vi "TCP.IP Server for Ripple Detection - Copy 3.vi"() -> ()   [LabVIEW 2021]
doc: "Demonstrates how to set up a basic TCP connection, send data to the specified port once a connection has been established, and terminate the connection once the data has been sent. This VI is designed to stop if the TCP connection is terminated. The data sent in this example is an array of random numbers."
panel:
  out "Waveform Graph 10":dbl[](graph)
  in  "loop 1":i32
  in  "Client Closed":string="The client VI closed the connection."
  in  "Stop":bool
  # "Overview: Demonstrates the use of the TCP functions to initialize a TCP server that can send data to a client VI.\nInstructions:\n1. Run the VI.\n2. Open Simple TCP - Client.vi and follow the instructions on its front panel. Note that if you wait longer than 30 seconds to do this after running this VI, it will time out.\n3. Click Stop to stop the VI. Note that if you stop the client VI, this VI will stop automatically."
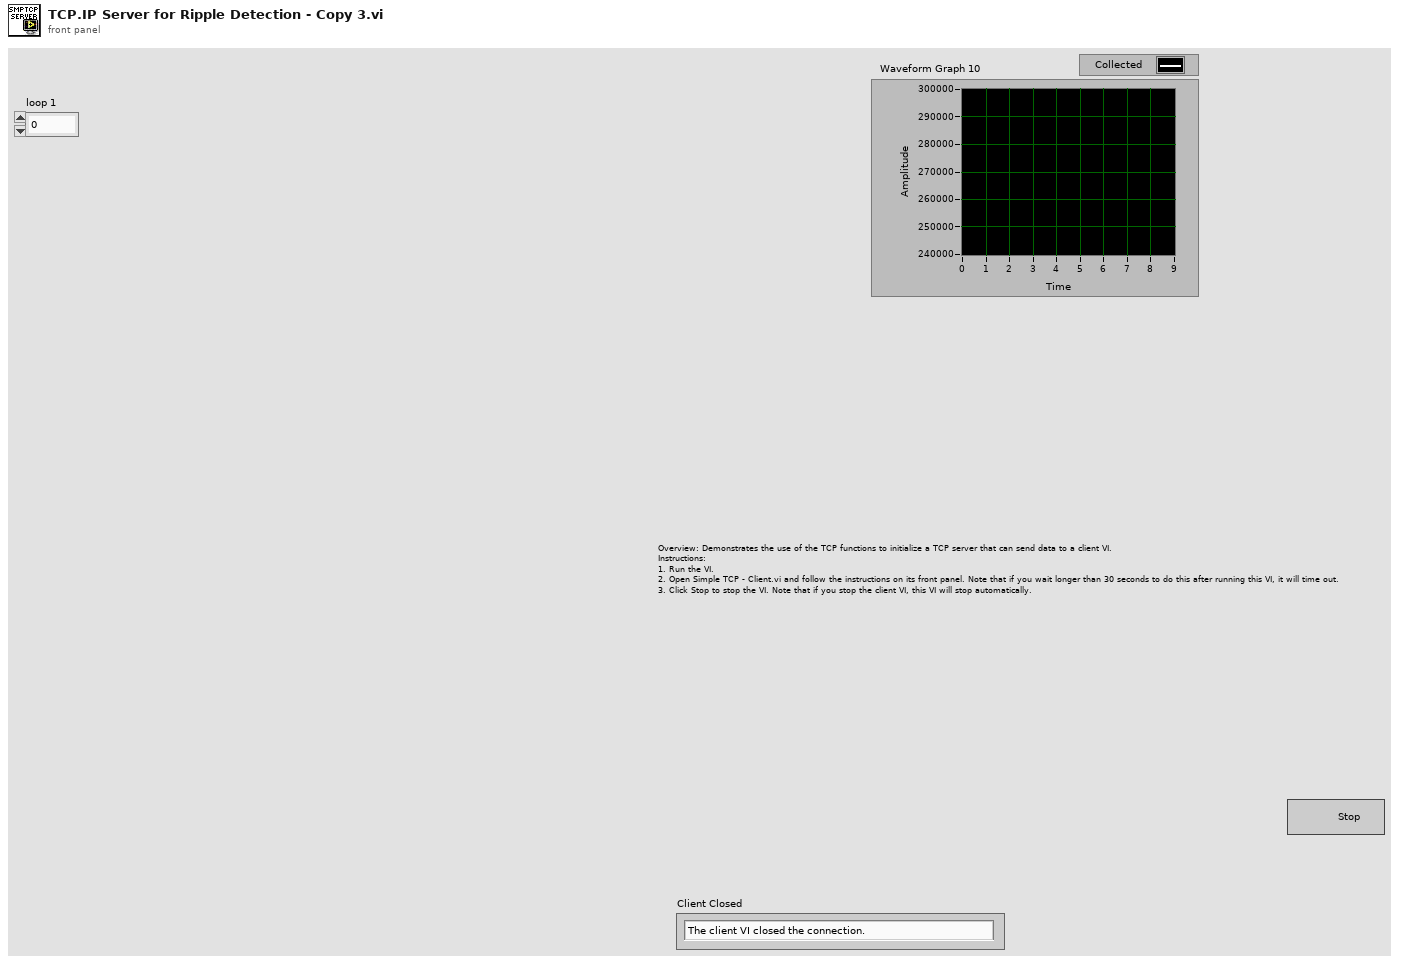
[diagram p1: front panel]
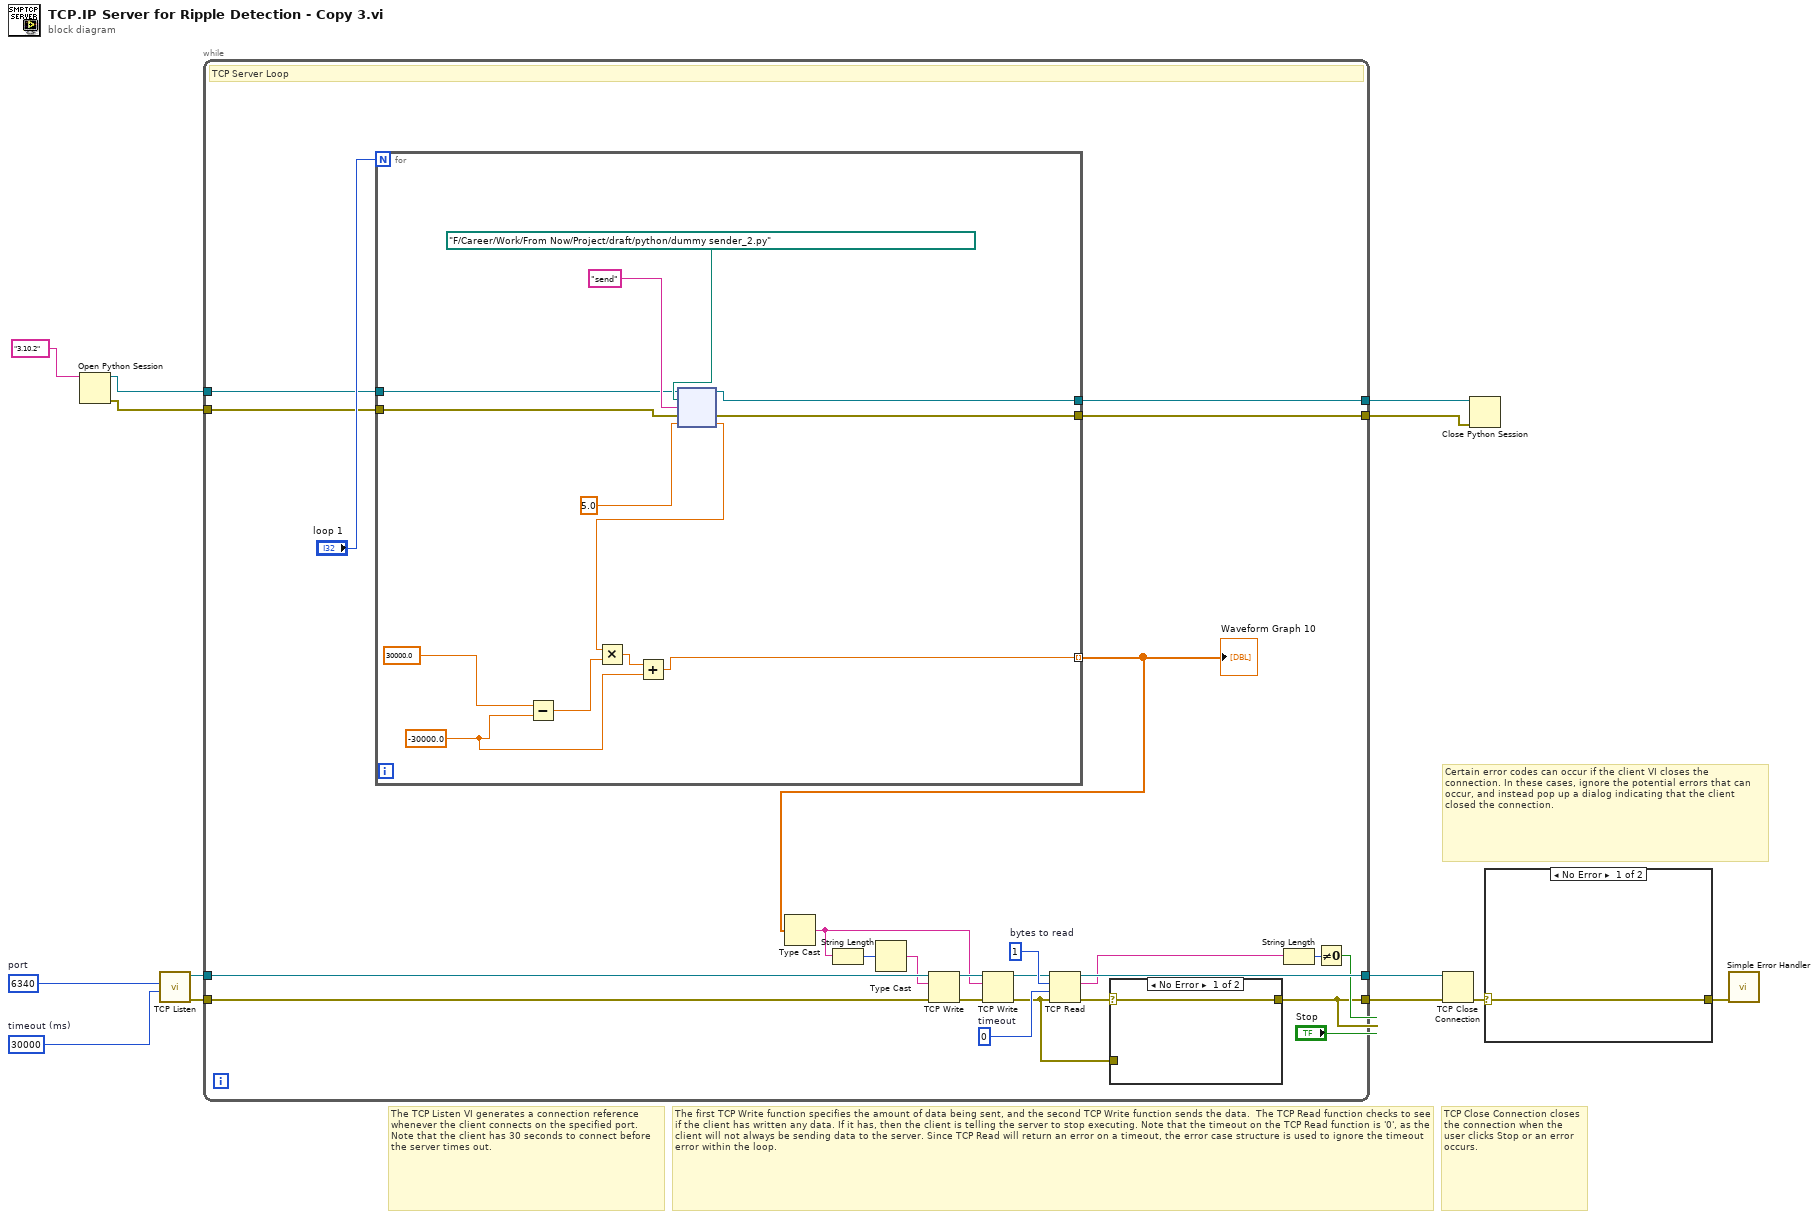
[diagram p0: block diagram]
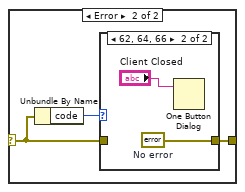
[diagram p2: hidden frame]
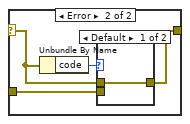
[diagram p4: hidden frame]
diagram:
  w6 = u16 6340  # port
  w7 = 30000  # timeout (ms)
  # "TCP Close Connection closes the connection when the user clicks Stop or an error occurs."
  # "The TCP Listen VI generates a connection reference whenever the client connects on the specified port. Note that the client has 30 seconds to connect before the server times out."
  # "Certain error codes can occur if the client VI closes the connection. In these cases, ignore the potential errors that can occur, and instead pop up a dialog indicating that the client closed the connection."
  # "The first TCP Write function specifies the amount of data being sent, and the second TCP Write function sends the data.  The TCP Read function checks to see if the client has written any data. If it has, then the client is telling the server to stop executing. Note that the timeout on the TCP Read function is '0', as the client will not always be sending data to the server. Since TCP Read will return an error on a timeout, the error case structure is used to ignore the timeout error within the loop."
  n1 = Open Python Session(python version="3.10.2" ("Python version")) -> (session out=w4:refnum<k35>, error out=w3:errorcluster)  [unwired: 2 in]
  n2 = call <vilib>:"TCP Listen.vi"("timeout ms (wait forever: -1)"=w7, "port"=w6) -> ("error out"=w8:errorcluster, "connection ID"=w9:refnum<k5>)  [unwired: 5 in, 3 out]
  n3 = while {
    tunnel: [w21] -> w12
    tunnel: [w27] -> w13
    tunnel: w9 -> [w38]
    tunnel: w8 -> [w31]
    tunnel: w4 -> [w17]
    tunnel: w3 -> [w16]
    tunnel: [w15] -> w2
    tunnel: [w14] -> w1
    stop <- w32 stop-if-true
    w26 = 0  # timeout
    w29 = 1  # bytes to read
    # "TCP Server Loop"
    n4 = for {
      N: "loop 1" -> [_]
      tunnel: [w43] -> w18 mode=indexing
      tunnel: w17 -> [w42]
      tunnel: w16 -> [w41]
      tunnel: [w40] -> w15
      tunnel: [w39] -> w14
      w48 = -30000.0 ("y")
      n5 = Subtract(x=30000.0, y=w48) -> (x-y=w51:dbl)
      n6 = node(w42, path "F:/Career/Work/From Now/Project/draft/python/dummy sender_2.py" ("module path"), "send" ("function name"), w41, 5.0) -> (w40:refnum<k35>, w39:errorcluster, w44:dbl)  [unwired: 2 out]
      n7 = Multiply(x=w44, y=w51) -> (x*y=w50:dbl)
      n8 = Add(x=w50, y=w48) -> (x+y=w43:dbl)
    }
    "Waveform Graph 10" <- w18
    n9 = Type Cast(x=w18) -> (*(type *) &x=w33:string)  [unwired: 1 out]
    n10 = String Length(string=w33) -> (length=w35:i32)
    n11 = Type Cast(x=w35) -> (*(type *) &x=w34:string)  [unwired: 1 out]
    n12 = TCP Write(connection ID=w38, data in=w34, error in (no error)=w31) -> (connection ID out=w37:refnum<k5>, error out=w36:errorcluster)  [unwired: 2 out]
    n13 = TCP Write(connection ID=w37, data in=w33, error in (no error)=w36) -> (connection ID out=w28:refnum<k5>, error out=w20:errorcluster)  [unwired: 2 out]
    n14 = TCP Read(connection ID=w28, bytes to read=w29, error in (no error)=w20, 9:w26) -> (connection ID out=w27:refnum<k5>, data out=w24:string, error out=w22:errorcluster)  [unwired: 1 out]
    n15 = case shown="No Error" w22 {
      selector: w22 -> [w52 w55]
      tunnel: [w52 w53] -> w21
      tunnel: w20 -> [_ w54]
      frame No Error {
      }
      frame Error {
        n16 = Unbundle By Name(w55) -> ("code"=w56:i32)
        n17 = case shown="Default" w56 {
          tunnel: w55 -> [w57 _]
          tunnel: w54 -> [_ w58]
          tunnel: [w57 w58] -> w53
          frame Default {
          }
          frame 56 {
          }
        }
      }
    }
    n18 = String Length(string=w24) -> (length=w25:i32)
    n19 = Not Equal To 0?(x=w25) -> (x != 0?=w23:bool)
    n20 = Compound Arithmetic op=OR(w23, w21, "Stop") -> (w32:bool)
  }
  n21 = TCP Close Connection(connection ID=w13, error in (no error)=w12) -> (error out=w11:errorcluster)  [unwired: 2 out]
  n22 = Close Python Session(session in=w2, error in=w1) -> ()  [unwired: 1 out]
  n23 = case shown="No Error" w11 {
    selector: w11 -> [w59 w61]
    tunnel: [w59 w60] -> w10
    frame No Error {
    }
    frame Error {
      n24 = Unbundle By Name(w61) -> ("code"=w62:i32)
      n25 = case shown="62, 64, 66" w62 {
        tunnel: w61 -> [w63 _]
        tunnel: [w63 w65] -> w60
        frame Default {
        }
        frame 62, 64, 66 {
          w65 = errorcluster {"status"=FALSE, "code"=0, "source"=""}  # No error
          n26 = One Button Dialog(message="Client Closed") -> ()  [unwired: 1 in, 1 out]
        }
      }
    }
  }
  n27 = call <vilib>:"Simple Error Handler.vi"("error in (no error)"=w10) -> ()  [unwired: 1 in, 8 out]
